vi "MasterReset.vi"(8 "error in (no error)":errorcluster, 11 "VISA Reference":refnum<visa-resource-name>) -> (0 "error out":errorcluster, 3 "dup VISA resource name":refnum<visa-resource-name>)   [LabVIEW 2016]
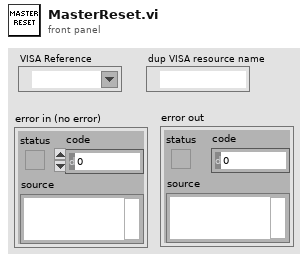
[diagram p1: front panel]
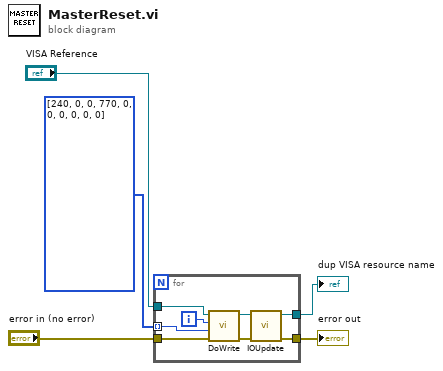
[diagram p0: block diagram]
diagram:
  n1 = for {
    tunnel: "VISA Reference" -> [w11]
    tunnel: "error in (no error)" -> [w10]
    tunnel: [w8] -> w2
    tunnel: [w9] -> w1
    tunnel: i32[] [240, 0, 0, 770, 0, 0, 0, 0, 0, 0] -> [w7] mode=indexing
    i -> [w6]
    n2 = call "DoWrite.vi"("error in (no error)"=w10, "Value"=w7, "Register Address"=w6, "VISA Reference"=w11) -> ("error out"=w12:errorcluster, "dup VISA resource name"=w13:refnum<visa-resource-name>)  [unwired: 6 in]
    n3 = call "IOUpdate.vi"("error in (no error)"=w12, "VISA Reference"=w13) -> ("error out"=w8:errorcluster, "dup VISA resource name"=w9:refnum<visa-resource-name>)  [unwired: 8 in]
  }
  "dup VISA resource name" <- w1
  "error out" <- w2
